vi "PololuTicMakeCommand.vi"(4 "ReadLength (bytes)":u8, 6 "Register":i32 format="%02x", 7 "VISA resource name":refnum<visa-resource-name>, 8 "errorIn":errorcluster, 10 "Argument":i32, 11 "PololuCommand":T1="FullScaleRatingSLPM") -> (0 "errorOut":errorcluster, 1 "Boolean array":bool[](array[boolean]) caption="LSB                                       MSB", 2 "32-bitReadValue":i32, 3 "read buffer":string)   [LabVIEW 2018]
uses:
  PololuCommand.ctl
panel:
  in  "ReplyType":enum16{"8-bit", "7-bit"}(ring)
  out "Command":string
  out "In Range?":bool
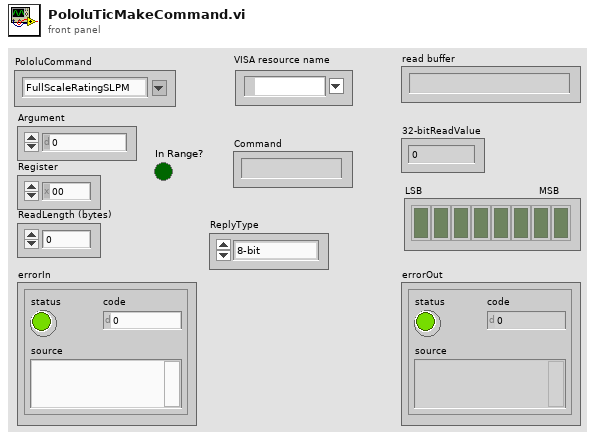
[diagram p1: front panel]
types:
  T1 = typedef "PololuCommand.ctl" = string
  T2 = typedef "PololuCommandDescriptor.ctl" = cluster{"PololuCommand":string, "Mnemonic":string, "CommandType":T3, "Min":i32, "Max":i32}
  T3 = typedef "TicCommandType.ctl" = enum16{"Command", "7-bitWrite", "32-bitWrite", "BlockRead"}
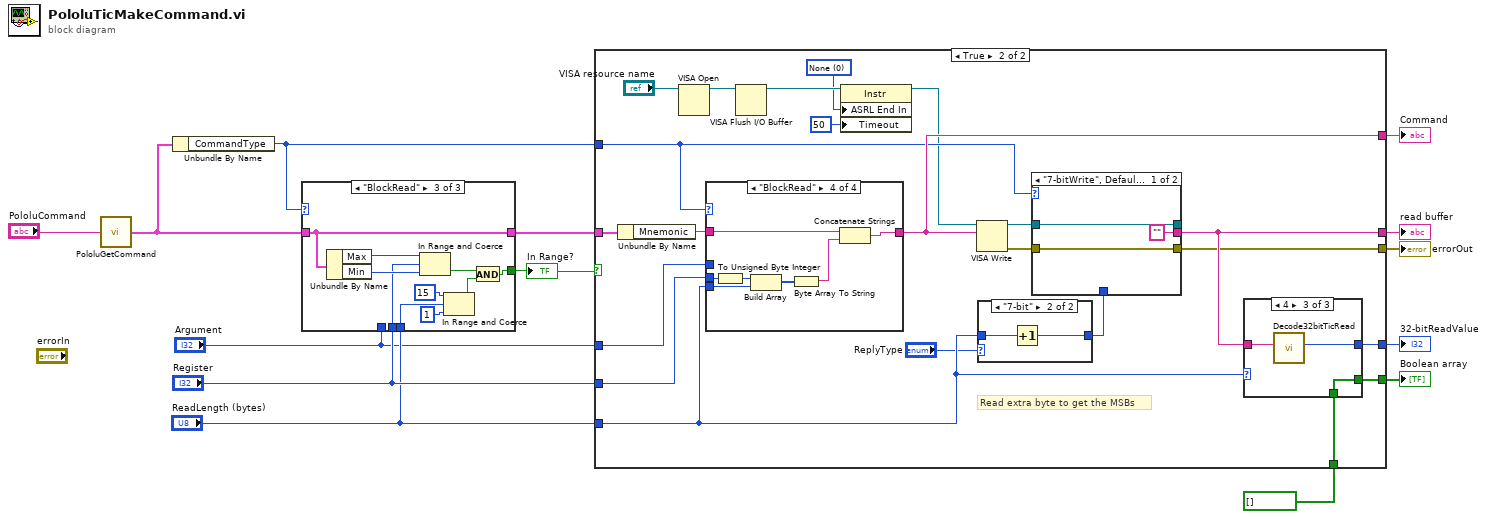
[diagram p0: block diagram]
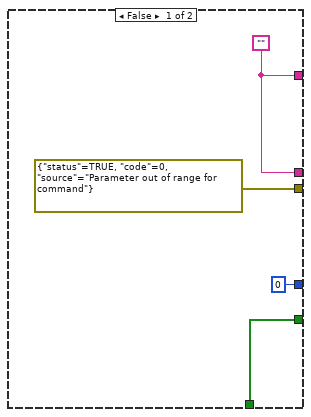
[diagram p2: hidden frame]
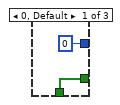
[diagram p4: hidden frame]
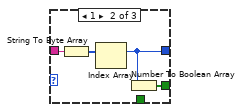
[diagram p5: hidden frame]
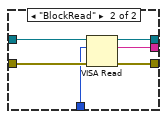
[diagram p6: hidden frame]
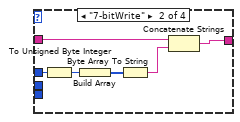
[diagram p8: hidden frame]
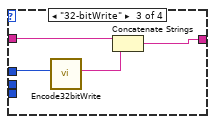
[diagram p9: hidden frame]
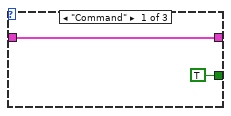
[diagram p10: hidden frame]
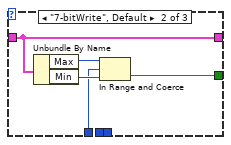
[diagram p11: hidden frame]
diagram:
  n1 = call "PololuGetCommand.vi"("PololuCommand"="PololuCommand") -> ("CommandDescriptor"=w13:T2)  [unwired: 3 in, 1 out]
  n2 = Unbundle By Name(w13) -> ("CommandType"=w9:T3)
  n3 = case shown="\"BlockRead\"" w9 {
    tunnel: [w16 w19 w28] -> w11
    tunnel: w13 -> [w16 w19 w28]
    tunnel: "Register" -> [_ _ w29]
    tunnel: [TRUE w18 w24] -> w1
    tunnel: "ReadLength (bytes)" -> [_ _ w27]
    tunnel: "Argument" -> [_ w17 _]
    frame "Command" {
    }
    frame "7-bitWrite", Default {
      n4 = Unbundle By Name(w19) -> ("Max"=w21:i32, "Min"=w20:i32)
      n5 = In Range and Coerce(upper limit=w21, x=w17, lower limit=w20) -> (In Range?=w18:bool)  [unwired: 1 out]
    }
    frame "BlockRead" {
      n6 = Unbundle By Name(w28) -> ("Max"=w31:i32, "Min"=w30:i32)
      n7 = In Range and Coerce(upper limit=w31, x=w29, lower limit=w30) -> (In Range?=w23:bool)  [unwired: 1 out]
      n8 = In Range and Coerce(upper limit=u8 15, x=w27, lower limit=u8 1) -> (In Range?=w22:bool)  [unwired: 1 out]
      n9 = And(x=w23, y=w22) -> (x .and. y?=w24:bool)
    }
  }
  "In Range?" <- w1
  n10 = case shown="True" w1 {
    tunnel: "Register" -> [_ w57]
    tunnel: w11 -> [_ w56]
    tunnel: [w32 w54] -> w10
    tunnel: w9 -> [_ w52]
    tunnel: [w32 w51] -> w8
    tunnel: [0 ("Value") w50] -> w7
    tunnel: "ReadLength (bytes)" -> [_ w49]
    tunnel: bool[] [] ("Boolean array") -> [w33 w48]
    tunnel: [w33 w47] -> w4
    tunnel: "Argument" -> [_ w46]
    tunnel: [errorcluster {"status"=TRUE, "code"=0, "source"="Parameter out of range for command"} ("error out") w44] -> w2
    frame False {
      w32 = ""
    }
    frame True {
      w39 = u16 0 items=["None", "Last Bit", "TermChar"] ("Serial Settings:End Mode for Reads")
      # "Read extra byte to get the MSBs"
      n11 = Unbundle By Name(w56) -> ("Mnemonic"=w55:string)
      n12 = VISA Open(VISA resource name="VISA resource name") -> (VISA resource name=w42:refnum<visa-resource-name>)  [unwired: 4 in, 1 out]
      n13 = case shown="\"BlockRead\"" w52 {
        tunnel: w57 -> [_ _ _ w96]
        tunnel: w55 -> [w79 w83 w89 w92]
        tunnel: [w79 w81 w87 w90] -> w54
        tunnel: w49 -> [_ _ _ w95]
        tunnel: w46 -> [_ w80 w86 _]
        frame "Command", Default {
        }
        frame "7-bitWrite" {
          n14 = To Unsigned Byte Integer(number=w80) -> (unsigned 8bit integer=w85:u8)
          n15 = Build Array(w85) -> (w84:u8[])
          n16 = Byte Array To String(unsigned byte array=w84) -> (string=w82:string)
          n17 = Concatenate Strings(w83, w82) -> (w81:string)
        }
        frame "32-bitWrite" {
          n18 = call "Encode32bitWrite.vi"("Numeric"=w86) -> ("PololuString"=w88:string)  [unwired: 10 in]
          n19 = Concatenate Strings(w89, w88) -> (w87:string)
        }
        frame "BlockRead" {
          n20 = To Unsigned Byte Integer(number=w96) -> (unsigned 8bit integer=w94:u8)
          n21 = Build Array(w94, w95) -> (w93:u8[])
          n22 = Byte Array To String(unsigned byte array=w93) -> (string=w91:string)
          n23 = Concatenate Strings(w92, w91) -> (w90:string)
        }
      }
      n24 = VISA Flush I/O Buffer(VISA resource name=w42) -> (VISA resource name out=w41:refnum<visa-resource-name>)  [unwired: 2 in, 1 out]
      n25 = property class="Instr"(reference=w41, "ASRL End In"=w39, "Timeout"=u32 50 ("General Settings:Timeout Value")) -> (reference out=w40:refnum<visa-resource-name>)  [unwired: 1 in, 1 out]
      n26 = VISA Write(VISA resource name=w40, write buffer=w54) -> (VISA resource name out=w53:refnum<visa-resource-name>, error out=w45:errorcluster)  [unwired: 1 in, 1 out]
      n27 = case shown="\"7-bit\"" "ReplyType" {
        tunnel: w49 -> [w58 w60]
        tunnel: [w58 w59] -> w37
        frame "8-bit", Default {
        }
        frame "7-bit" {
          n28 = Increment(x=w60) -> (x+1=w59:u8)
        }
      }
      n29 = case shown="\"7-bitWrite\", Default" w52 {
        tunnel: w53 -> [w70 w78]
        tunnel: ["" ("read buffer") w77] -> w51
        tunnel: w45 -> [w71 w76]
        tunnel: [w71 w75] -> w44
        tunnel: [w70 w74] -> _
        tunnel: w37 -> [_ w73]
        frame "7-bitWrite", Default {
        }
        frame "BlockRead" {
          n30 = VISA Read(VISA resource name=w78, byte count=w73, error in (no error)=w76) -> (VISA resource name out=w74:refnum<visa-resource-name>, read buffer=w77:string, error out=w75:errorcluster)  [unwired: 1 out]
        }
      }
      n31 = case shown="4" w49 {
        tunnel: w51 -> [_ w66 w69]
        tunnel: [0 ("Value") w64 w68] -> w50
        tunnel: [w61 w63 w67] -> w47
        tunnel: w48 -> [w61 _ w67]
        frame 0, Default {
        }
        frame 1 {
          n32 = String To Byte Array(string=w66) -> (unsigned byte array=w65:u8[])
          n33 = Index Array(array=w65) -> (element=w64:u8)  [unwired: 1 in]
          n34 = Number To Boolean Array(number=w64) -> (Boolean array=w63:bool[])
        }
        frame 4 {
          n35 = call "Decode32bitTicRead.vi"("ReadHex"=w69) -> ("Value"=w68:i32)  [unwired: 10 in]
        }
      }
    }
  }
  "Command" <- w10
  "read buffer" <- w8
  "32-bitReadValue" <- w7
  "Boolean array" <- w4
  "errorOut" <- w2
